vi "GEA2 Initialize.vi"(0 "Board Index":i32, 5 "Source Address":u8=228 format="%.0x", 11 "error in":errorcluster) -> (4 "GEA2 Reference Out":refnum<k24>, 8 "Board ID":string, 15 "error out":errorcluster)   [LabVIEW 2019, in "GEA2_Toolkit.lvlib"]
doc: "This VI uses .NET DLLs to initialize a GEA2 connection over USB. The output is a reference to the newly opened GEA2 connection."
uses:
  library/GEA2_Toolkit.lvlib
  C:/TechnologyLab/NI-2010/Drivers/GEA3 Toolkit/GEA3 DLL Source/GeaCommunication.dll
  GEA3 DLL Source/GeaCommunication.dll
panel:
  in  "IPC?":bool
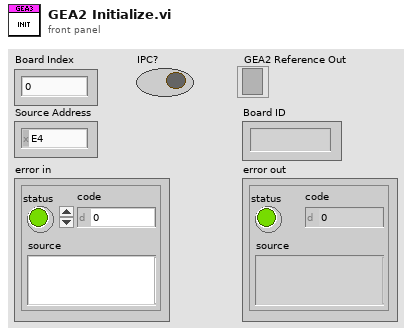
[diagram p1: front panel]
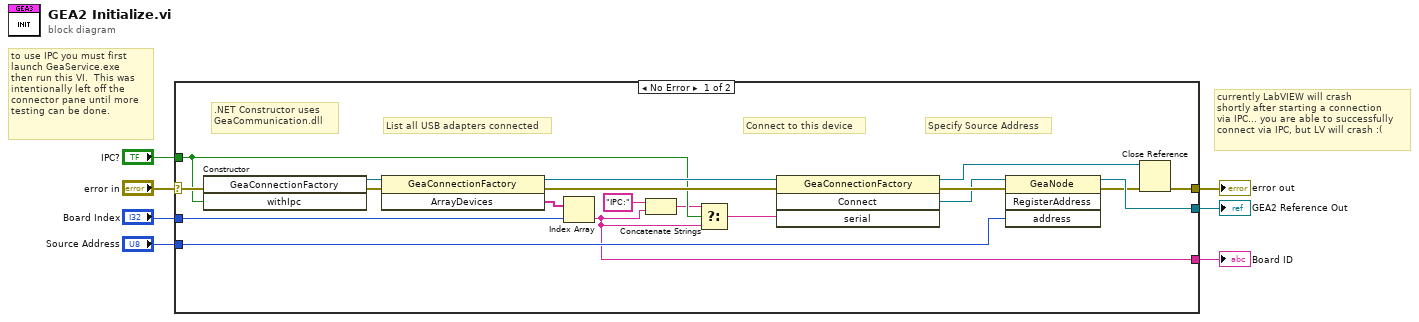
[diagram p0: block diagram]
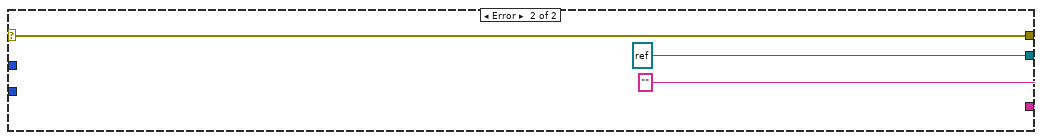
[diagram p2: hidden frame]
diagram:
  # "currently LabVIEW will crash\nshortly after starting a connection\nvia IPC... you are able to successfully\nconnect via IPC, but LV will crash :("
  # "to use IPC you must first\nlaunch GeaService.exe\nthen run this VI.  This was\nintentionally left off the\nconnector pane until more\ntesting can be done."
  n1 = case shown="No Error" "error in" {
    selector: "error in" -> [w21 w29]
    tunnel: "Board Index" -> [w16 _]
    tunnel: [w14 w29] -> w7
    tunnel: [w24 refnum<k24> refnum ("Connect")] -> w5
    tunnel: "Source Address" -> [w22 _]
    tunnel: [w9 "" ("get_Item")] -> w2
    tunnel: "IPC?" -> [w12 _]
    frame No Error {
      # "Specify Source Address"
      # "Connect to this device"
      # "List all USB adapters connected"
      # ".NET Constructor uses\nGeaCommunication.dll"
      n2 = constructor class="GeaConnectionFactory"(error in=w21, "withIpc"=w12) -> (reference out=w13:refnum<k24>, error out=w20:errorcluster)  [unwired: 2 in, 2 out]
      n3 = invoke class="GeaConnectionFactory" method="ArrayDevices"(reference=w13, error in=w20) -> (reference out=w19:refnum<k24>, error out=w15:errorcluster, "ArrayDevices"=w17:string[])  [unwired: 1 in]
      n4 = Index Array(array=w17, index=w16) -> (element=w9:string)
      n5 = Concatenate Strings("IPC:" ("string"), w9) -> (w8:string)
      n6 = Select(t=w8, s=w12, f=w9) -> (s? t:f=w10:string)
      n7 = invoke class="GeaConnectionFactory" method="Connect"(reference=w19, error in=w15, "serial"=w10) -> (reference out=w25:refnum<k24>, error out=w26:errorcluster, "Connect"=w18:refnum<k24>)  [unwired: 1 in, 1 out]
      n8 = invoke class="GeaNode" method="RegisterAddress"(reference=w18, error in=w26, "address"=w22) -> (reference out=w24:refnum<k24>, error out=w23:errorcluster)  [unwired: 1 in, 2 out]
      n9 = Close Reference(reference=w25, error in (no error)=w23) -> (error out=w14:errorcluster)
    }
    frame Error {
    }
  }
  "error out" <- w7
  "GEA2 Reference Out" <- w5
  "Board ID" <- w2
